vi "Signal Generation.vi"(0 "Output Fs":dbl, 1 "Filter":bool, 2 "Low cutoff":dbl=20.0 format="%#_13g", 3 "High cutoff":dbl=20000.0 format="%#_13g", 5 "Signal Type":T1, 7 "Frequency 1":dbl, 9 "Frequency 2":dbl, 11 "Samples":dbl, 12 "File path":path) -> (6 "Output Signal":dbl[](array[numeric]))   [LabVIEW 2016]
uses:
  Modulation_Signals.ctl
  <vilib>/Analysis/3filter.llb/Filter Passband Type.ctl
  <vilib>/Waveform/WDTOps.llb/WDT Get Waveform Subset DBL.vi
  <vilib>/measure/maresamp.llb/Resample Waveform (single shot).vi
  <vilib>/Analysis/3filter.llb/Butterworth Filter (DBL).vi
  <vilib>/Analysis/NI_AALBase.lvlib
  <vilib>/measure/NI_MAPro.lvlib
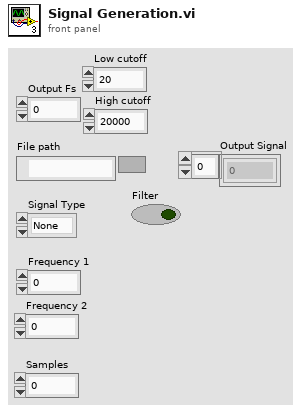
[diagram p1: front panel]
types:
  T1 = typedef "Modulation_Signals.ctl" = enum16{"None", "Sine", "Chirp", "White Noise", "File"}
  T2 = typedef "NI_AALBase.lvlib/Filter Passband Type.ctl" = enum32{"Lowpass", "Highpass", "Bandpass", "Bandstop"}
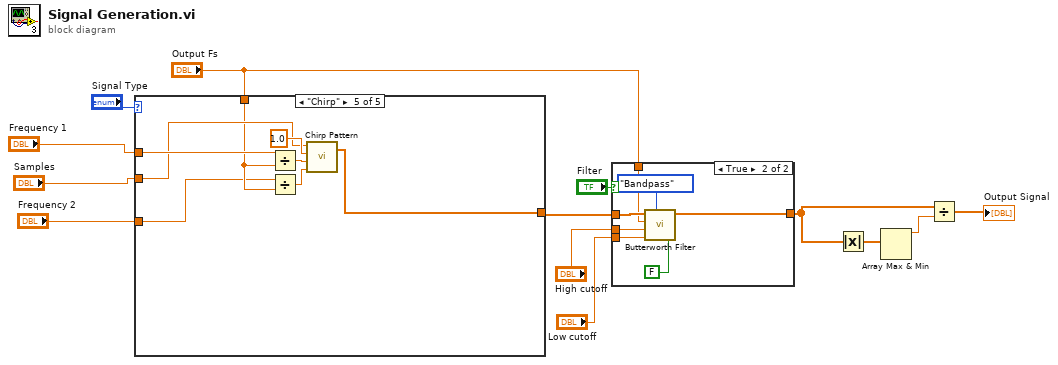
[diagram p0: block diagram]
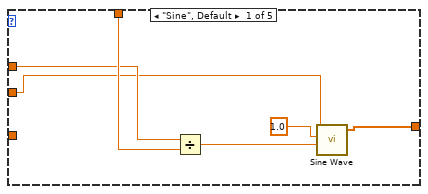
[diagram p3: hidden frame]
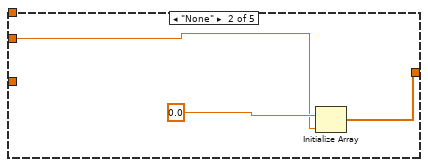
[diagram p4: hidden frame]
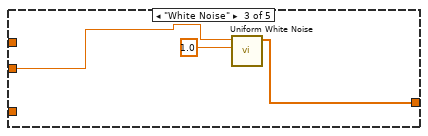
[diagram p5: hidden frame]
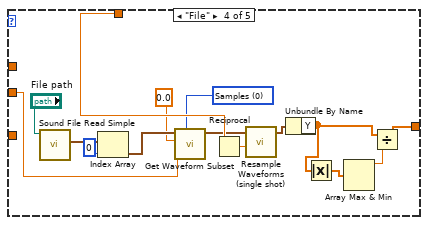
[diagram p6: hidden frame]
diagram:
  n1 = case shown="\"Chirp\"" "Signal Type" {
    tunnel: [w17 w21 w24 w29 w48] -> w10
    tunnel: "Output Fs" -> [w16 _ _ w37 w44]
    tunnel: "Frequency 1" -> [w15 _ _ _ w46]
    tunnel: "Samples" -> [w14 w20 w23 w26 w45]
    tunnel: "Frequency 2" -> [_ _ _ _ w43]
    frame "Sine", Default {
      n2 = Divide(x=w15, y=w16) -> (x/y=w18:dbl)
      n3 = call <vilib>:"Sine Wave.vi"("samples"=w14, "amplitude"=1.0, "frequency"=w18) -> ("sine wave"=w17:dbl[])  [unwired: 2 in, 2 out]
    }
    frame "None" {
      n4 = Initialize Array(0.0 ("element"), w20) -> (w21:dbl[])
    }
    frame "White Noise" {
      n5 = call <vilib>:"Uniform White Noise.vi"("amplitude"=1.0, "samples"=w23) -> ("uniform white noise"=w24:dbl[])  [unwired: 8 in, 1 out]
    }
    frame "File" {
      w34 = u16 0 items=["Samples", "Relative Time"] ("start/duration format")
      n6 = call <vilib>:"Sound File Read Simple.vi"("path"="File path") -> ("data"=w36:waveform(dbl)[])  [unwired: 7 in, 3 out]
      n7 = Index Array(array=w36, index=0) -> (element=w35:waveform(dbl))
      n8 = call-poly <vilib>:"Get Waveform Subset.vi"("start/duration format"=w34, "duration"=w26, "start samples/time"=0.0, "waveform in"=w35) -> ("waveform out"=w32:waveform(dbl))  [unwired: 2 in, 3 out]
      n9 = Reciprocal(x=w37) -> (1/x=w39:dbl)
      n10 = call-poly <vilib>:"Resample Waveforms (single shot).vi"("waveform in"=w32, "dt"=w39) -> ("resampled waveform out"=w31:waveform(dbl))  [unwired: 10 in, 3 out]
      n11 = Unbundle By Name(w31) -> ("Y"=w28:dbl[])
      n12 = Absolute Value(x=w28) -> (abs(x)=w27:dbl[])
      n13 = Array Max & Min(array=w27) -> (max value=w30:dbl)  [unwired: 3 out]
      n14 = Divide(x=w28, y=w30) -> (x/y=w29:dbl[])
    }
    frame "Chirp" {
      n15 = Divide(x=w46, y=w44) -> (x/y=w42:dbl)
      n16 = Divide(x=w43, y=w44) -> (x/y=w41:dbl)
      n17 = call <vilib>:"Chirp Pattern.vi"("f2"=w41, "f1"=w42, "amplitude"=1.0, "samples"=w45) -> ("Chirp Pattern"=w48:dbl[])  [unwired: 1 out]
    }
  }
  n18 = case shown="True" "Filter" {
    tunnel: w10 -> [w49 w56]
    tunnel: "Low cutoff" -> [_ w55]
    tunnel: "High cutoff" -> [_ w54]
    tunnel: "Output Fs" -> [_ w53]
    tunnel: [w49 w51] -> w2
    frame False {
    }
    frame True {
      n19 = call-poly <vilib>:"Butterworth Filter.vi"("init/cont (init:F)"=FALSE, "filter type"=Filter_Passband_Type."Bandpass", "low cutoff freq: fl"=w55, "high cutoff freq: fh"=w54, "sampling freq: fs"=w53, "X"=w56) -> ("Filtered X"=w51:dbl[])  [unwired: 2 in, 1 out]
    }
  }
  n20 = Absolute Value(x=w2) -> (abs(x)=w4:dbl[])
  n21 = Array Max & Min(array=w4) -> (max value=w3:dbl)  [unwired: 3 out]
  n22 = Divide(x=w2, y=w3) -> (x/y=→"Output Signal":dbl[])
